vi "Main.vi"(11 "Module Admin":refnum<class "Delacor_lib_QMH_Module Admin.lvclass">) -> ()   [LabVIEW 2020, in "UART Module.lvlib"]
doc: "This template is based off of the Queued Message Handler design pattern and the Queued Message Handler project template that ships with LabVIEW.\n\nThe main difference is that the queue is private to this module and communication between modules is performed via Broadcast and Request events.\n\nRequest events are wrapped in public API methods and are handled in the Event Handling Loop (EHL) of this VI. Any module can register for Broadcast events sent by this module. The EHL generates messages based on user interface actions.\n\nThe Message Handling Loop (MHL) processes messages generated by the EHL, or by other messages. The messages are string values, so new messages can be added easily to the Message Cases case structure in the MHL. Each message cluster can also provide an optional value for Message Data, which is a variant that can be converted to whatever message-specific data is required.\n_____\nBased on DQMH Project Template 7.0.1.1316."
uses:
  UART Module.lvlib
  <vilib>/Delacor/Delacor QMH/Libraries/Module Admin_class/Delacor_lib_QMH_Module Admin.lvclass
  Module Data--cluster.ctl
  Stop Argument--cluster.ctl
  <vilib>/Delacor/Delacor QMH/Libraries/Message Queue_class/Delacor_lib_QMH_Message Queue.lvclass/Delacor_lib_QMH_Message Queue.ctl
  <vilib>/Delacor/Delacor QMH/Libraries/Module Admin_class/Delacor_lib_QMH_Module Admin.lvclass/Delacor_lib_QMH_Module Admin.ctl
  Open Port Argument--cluster.ctl
  Close Port Argument--cluster.ctl
  <vilib>/Utility/miscctls.llb/LVPointTypeDef.ctl
  <vilib>/Delacor/Delacor QMH/Libraries/Message Queue_class/Delacor_lib_QMH_Enqueue Message (Single).vi
  <vilib>/Delacor/Delacor QMH/Libraries/Module Admin_class/Delacor_lib_QMH_Get External Launch.vi
  <vilib>/Delacor/Delacor QMH/Libraries/Message Queue_class/Delacor_lib_QMH_Message Queue.lvclass
  Write Data Argument--cluster.ctl
  checkBufferData Argument--cluster.ctl
  readBuffer Argument--cluster.ctl
  cc7c8281-b699-4288-b638-b774a9bc16a2.vi
  checkBufferSize Argument--cluster.ctl
panel:
  in  "stop":bool
  in  "讀取目標字數":i32=1
  in  "Write":bool
  in  "VISA resource name":refnum<visa-resource-name>
  out "read buffer":string
  in  "write buffer":string
  out "error out":errorcluster
  # "1. 設定 VISA\n2. 設定讀取目標字數\n3. 按下”開始通訊”，進行通訊作業\n4. 設定\"write buffer“\n5. 按下\"Write\"，將資料進行寫入\n6. 觀察\"read buffer\"\n7. 按下停止通訊“，結束通訊作業"
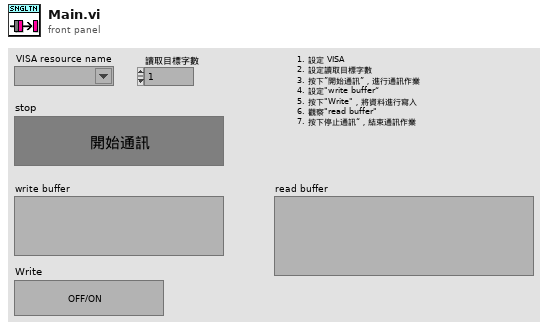
[diagram p1: front panel]
types:
  T1 = typedef "UART Module.lvlib/Request Events--cluster.ctl" = cluster{"Stop Module":refnum<user-event>, "Show Panel":refnum<user-event>, "Hide Panel":refnum<user-event>, "Get Module Execution Status":refnum<user-event>, "Show Diagram":refnum<user-event>, "Open Port":refnum<user-event>, "Close Port":refnum<user-event>, "Write Data":refnum<user-event>, "Private":cluster{"checkBufferData":refnum<user-event>, "readBuffer":refnum<user-event>, "checkBufferSize":refnum<user-event>}}
  T2 = typedef "UART Module.lvlib/Module Data--cluster.ctl" = cluster{"Status":string, "read buffer":string, "VISA":refnum<visa-resource-name>, "targetCount":i32}
  T3 = enum32{"invalid lock state", "Not Locked", "Locked (No Password)", "Password-protected"}
  T4 = typedef "UART Module.lvlib/Stop Argument--cluster.ctl" = cluster{"Origin":string, "Exit via Stop Module Req?":bool, "Wait for Module to stop?":bool}
  T5 = typedef "UART Module.lvlib/Open Port Argument--cluster.ctl" = cluster{"VISA":refnum<visa-resource-name>}
  T6 = typedef "UART Module.lvlib/Close Port Argument--cluster.ctl" = cluster{"Boolean":bool}
  T7 = typedef "UART Module.lvlib/Write Data Argument--cluster.ctl" = cluster{"write data":string}
  T8 = typedef "UART Module.lvlib/checkBufferData Argument--cluster.ctl" = cluster{"Boolean":bool}
  T9 = typedef "UART Module.lvlib/readBuffer Argument--cluster.ctl" = cluster{"Number of Bytes at Serial Port":u32}
  T10 = typedef "UART Module.lvlib/checkBufferSize Argument--cluster.ctl" = cluster{"readBuffer":string}
  T11 = typedef "LVPointTypeDef.ctl" = cluster{"Horizontal":i16, "Vertical":i16}
  T12 = enum32{"Invalid", "Standard", "Closed", "Hidden", "Minimized", "Maximized"}
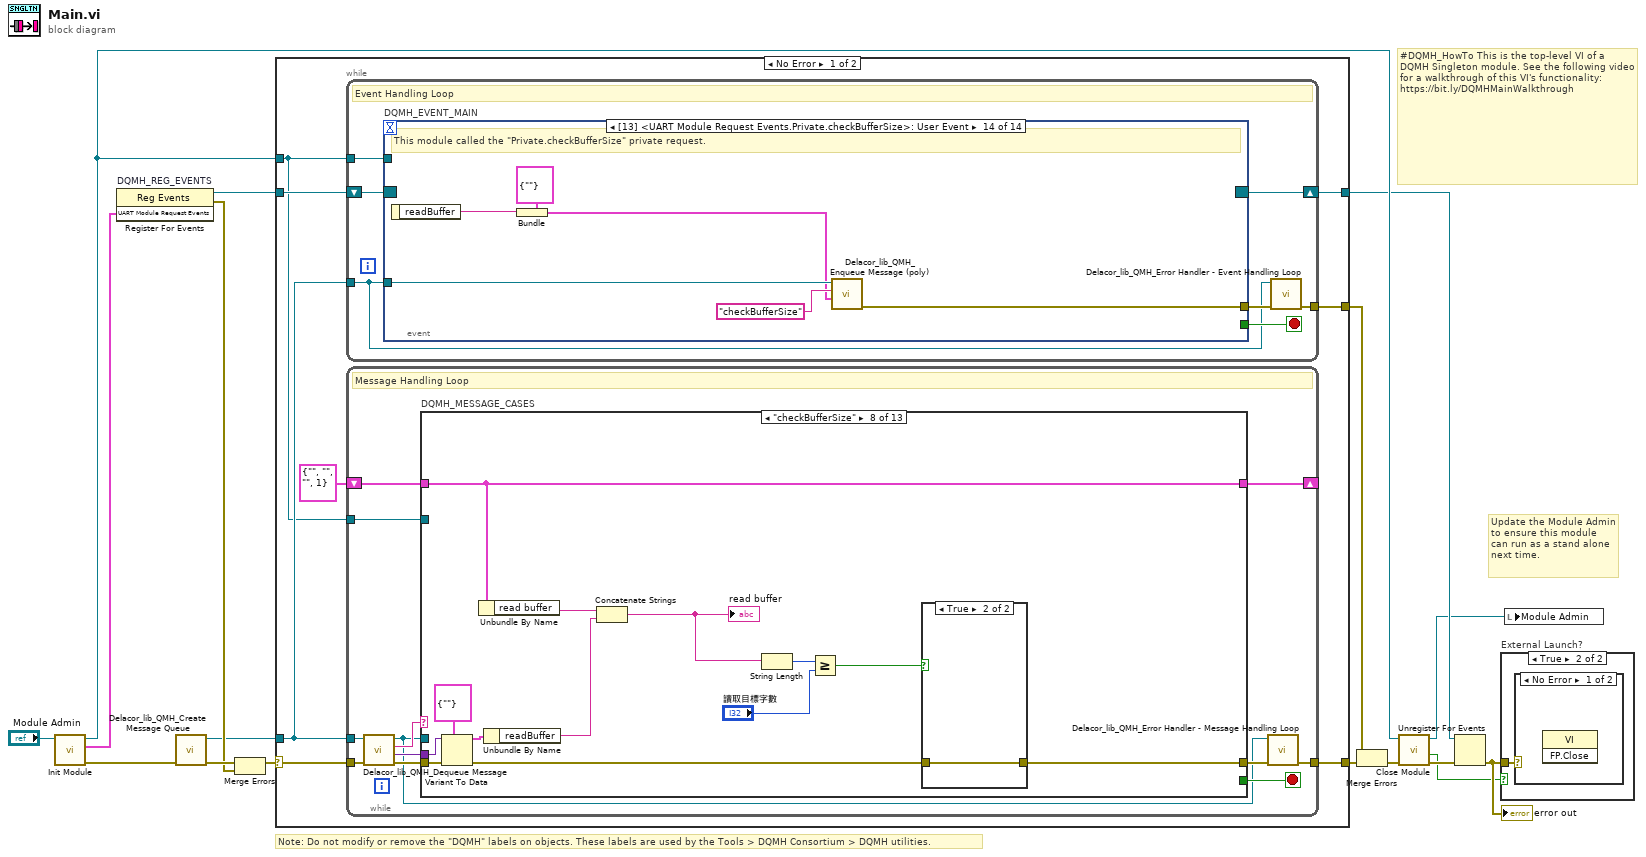
[diagram p0: block diagram]
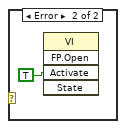
[diagram p3: hidden frame]
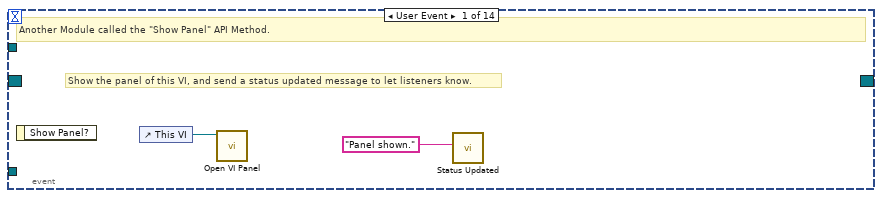
[diagram p4: hidden frame]
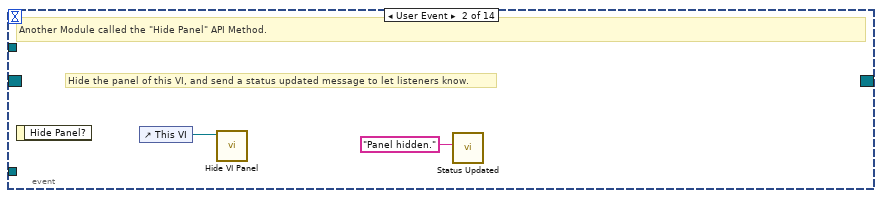
[diagram p5: hidden frame]
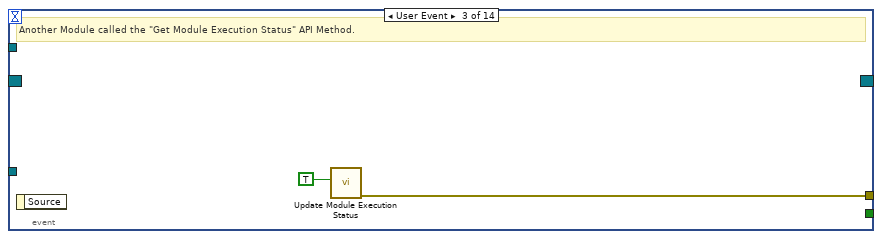
[diagram p6: hidden frame]
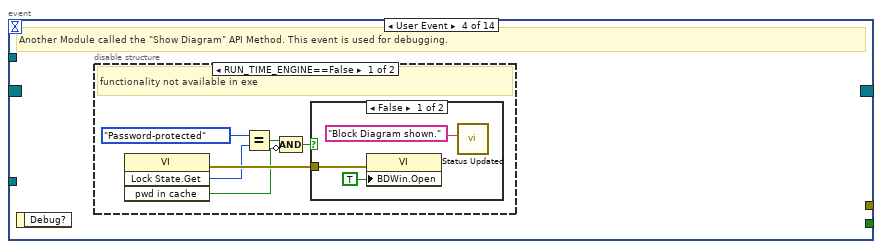
[diagram p7: hidden frame]
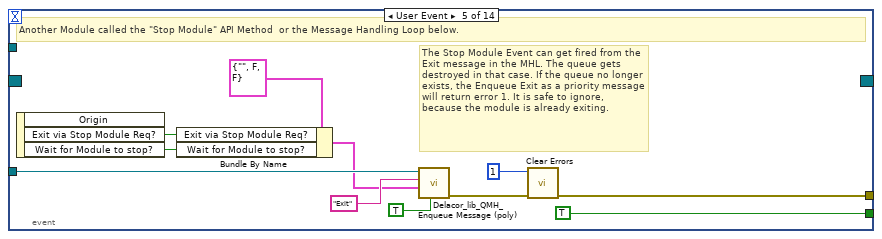
[diagram p10: hidden frame]
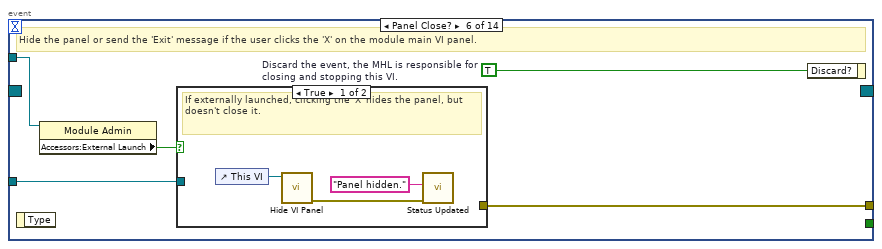
[diagram p11: hidden frame]
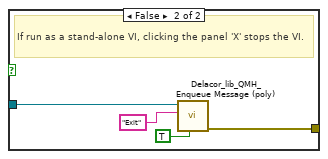
[diagram p12: hidden frame]
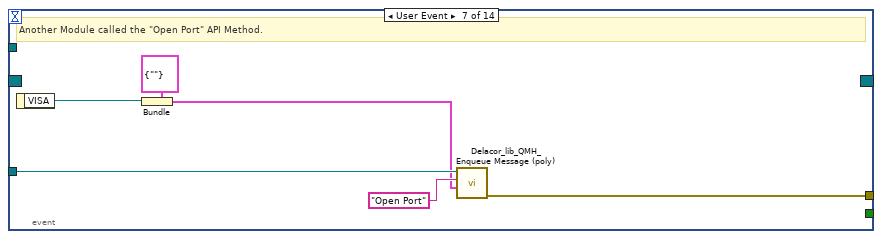
[diagram p13: hidden frame]
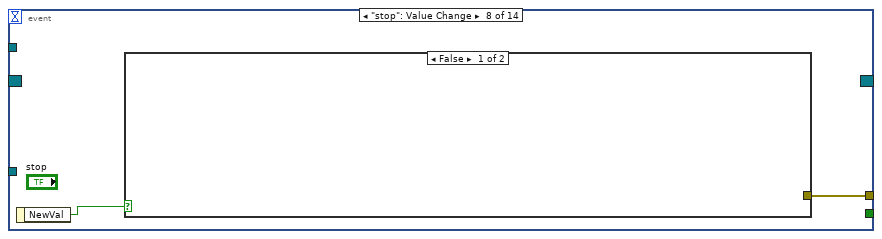
[diagram p14: hidden frame]
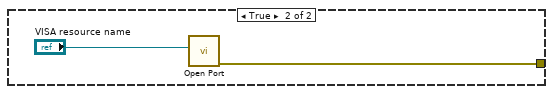
[diagram p15: hidden frame]
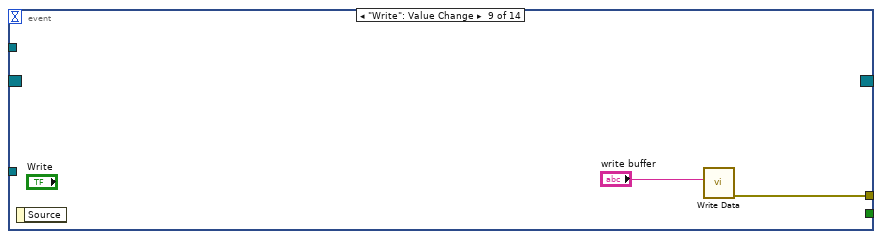
[diagram p16: hidden frame]
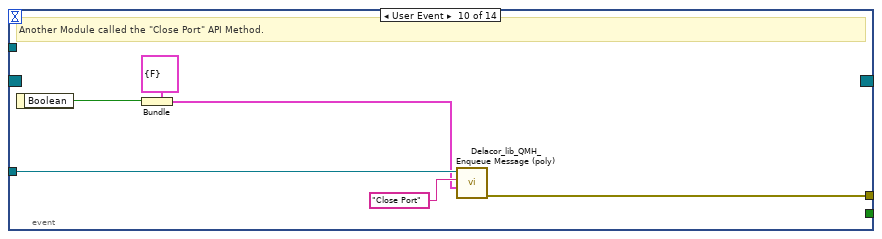
[diagram p17: hidden frame]
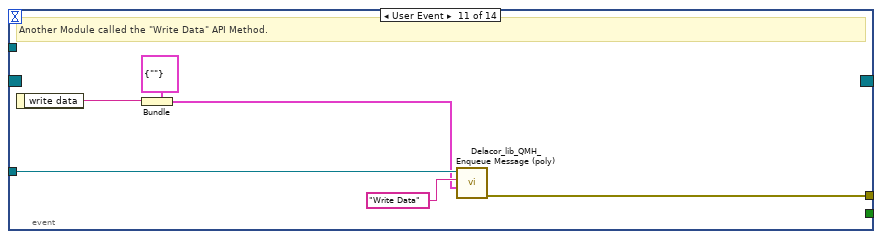
[diagram p18: hidden frame]
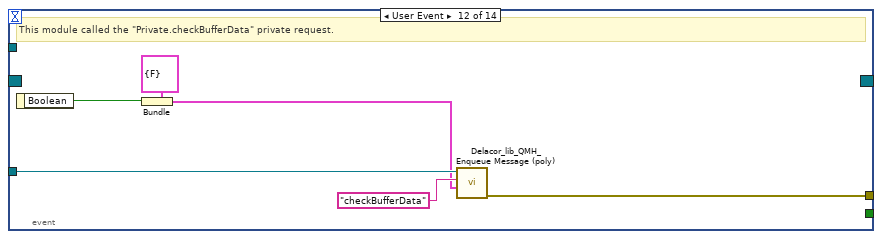
[diagram p19: hidden frame]
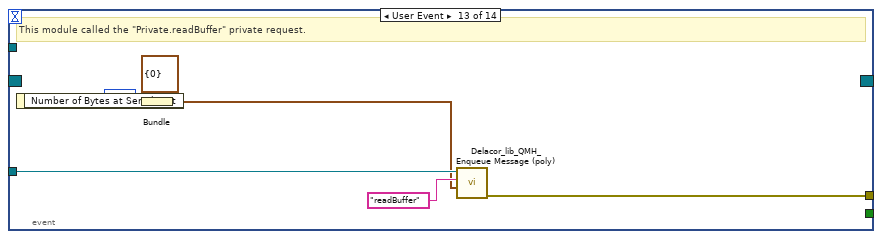
[diagram p20: hidden frame]
diagram:
  # "#DQMH_HowTo This is the top-level VI of a DQMH Singleton module. See the following video for a walkthrough of this VI's functionality: https://bit.ly/DQMHMainWalkthrough"
  # "Note: Do not modify or remove the \"DQMH\" labels on objects. These labels are used by the Tools > DQMH Consortium > DQMH utilities."
  # "Update the Module Admin to ensure this module can run as a stand alone next time."
  n1 = call "Init Module.vi"("Singleton Module Admin in"="Module Admin") -> ("error out"=w16:errorcluster, "UART Module Request Events"=w5:T1, "Singleton Module Admin out"=w8:refnum<class "Delacor_lib_QMH_Module Admin.lvclass">)  [unwired: 8 in]
  n2 = register-events "DQMH_REG_EVENTS"(w5) -> (reference out=w6:refnum<event-registration>, error out=w9:errorcluster)  [unwired: 2 in]
  n3 = call <vilib>:"Delacor_lib_QMH_Create Message Queue.vi"("error in"=w16) -> ("error out"=w11:errorcluster, "Message Queue"=w4:refnum<class "Delacor_lib_QMH_Message Queue.lvclass">)  [unwired: 9 in]
  n4 = Merge Errors(w11, w9) -> (w10:errorcluster)
  n5 = case shown="No Error" w10 {
    selector: w10 -> [w23 w276]
    tunnel: [w25 w275] -> w17
    tunnel: [w22 w274] -> w7
    tunnel: w6 -> [w20 w274]
    tunnel: w4 -> [w19 w269]
    tunnel: [w24 _] -> w14
    tunnel: w8 -> [w18 w270]
    frame No Error {
      n6 = while {
        tunnel: w19 -> [w26]
        shift-right: [w29] -> w22
        shift-left: w20 -> [w30]
        tunnel: [w31] -> w24
        tunnel: w18 -> [w27]
        stop <- w28 stop-if-true
        # "Event Handling Loop"
        n7 = event "DQMH_EVENT_MAIN" shown="[13] <UART Module Request Events.Private.checkBufferSize>: User Event" {
          selector: w30 -> [_ _ _ _ _ _ _ _ _ _ _ _ _ _]
          dyn-events: [_ _ _ _ _ _ _ _ _ _ _ _ _ _] -> w29
          timeout: _ -> [_ _ _ _ _ _ _ _ _ _ _ _ _ _]
          tunnel: [_ _ _ _ TRUE ("Discard?") _ _ _ _ _ _ _ _ _] -> w28
          tunnel: w26 -> [_ _ _ _ w54 w61 w76 _ _ w88 w94 w100 w106 w112]
          tunnel: [_ _ w38 _ w57 w63 w71 w77 w82 w83 w89 w95 w101 w107] -> w32
          tunnel: w27 -> [_ _ _ _ _ w60 _ _ _ _ _ _ _ _]
          event User Event {
            # "Show the panel of this VI, and send a status updated message to let listeners know."
            # "Another Module called the \"Show Panel\" API Method."
            n8 = event-data() -> ()  [unwired: 1 in, 1 out]
            n9 = control-ref of="This VI"() -> (w34:refnum<vi>)
            n10 = call "Open VI Panel.vi"("VI"=w34) -> ()  [unwired: 10 in, 1 out]
            n11 = call "Status Updated.vi"("Status"="Panel shown." ("format string")) -> ()  [unwired: 10 in, 1 out]
          }
          event User Event {
            # "Hide the panel of this VI, and send a status updated message to let listeners know."
            # "Another Module called the \"Hide Panel\" API Method."
            n12 = event-data() -> ()  [unwired: 1 in, 1 out]
            n13 = control-ref of="This VI"() -> (w36:refnum<vi>)
            n14 = call "Hide VI Panel.vi"("VI"=w36) -> ()  [unwired: 10 in, 1 out]
            n15 = call "Status Updated.vi"("Status"="Panel hidden." ("format string")) -> ()  [unwired: 10 in, 1 out]
          }
          event User Event {
            # "Another Module called the \"Get Module Execution Status\" API Method."
            n16 = event-data() -> ()  [unwired: 1 in, 1 out]
            n17 = call "Update Module Execution Status.vi"("Running?"=TRUE) -> ("error out"=w38:errorcluster)  [unwired: 10 in]
          }
          event User Event {
            # "Another Module called the \"Show Diagram\" API Method. This event is used for debugging."
            n18 = event-data() -> ()  [unwired: 1 in, 1 out]
            n19 = disable-structure shown="RUN_TIME_ENGINE==False" {
              frame condition #0 (active) {
                # "functionality not available in exe"
                n20 = invoke on="Invoke Node" class="VI" method="Lock State.Get"() -> (error out=w44:errorcluster, "Get Lock State"=w43:T3, "pwd in cache"=w40:bool)  [unwired: 4 in, 1 out]
                n21 = Equal?(x=T3."Password-protected", y=w43) -> (x = y?=w41:bool)
                n22 = Compound Arithmetic op=AND(w41, invert w40) -> (w39:bool)
                n23 = case shown="False" w39 {
                  tunnel: w44 -> [w47 _]
                  frame False {
                    n24 = property on="Property Node" class="VI"(error in=w47, "BDWin.Open"=TRUE ("Block Diagram Window:Open")) -> ()  [unwired: 1 in, 2 out]
                    n25 = call "Status Updated.vi"("Status"="Block Diagram shown." ("format string")) -> ()  [unwired: 10 in, 1 out]
                  }
                  frame True {
                    # "Password-protected VI, and the password is not in the cache. Do not show the diagram."
                  }
                }
              }
              frame condition #1 {
              }
            }
          }
          event User Event {
            # "The Stop Module Event can get fired from the Exit message in the MHL. The queue gets destroyed in that case. If the queue no longer exists, the Enqueue Exit as a priority message will return error 1. It is safe to ignore, because the module is already exiting."
            # "Another Module called the \"Stop Module\" API Method  or the Message Handling Loop below."
            n26 = event-data() -> ("Exit via Stop Module Req?"=w50:bool, "Wait for Module to stop?"=w49:bool)  [unwired: 1 in, 1 out]
            n27 = Bundle By Name(cluster=T4 {"Origin"="", "Exit via Stop Module Req?"=FALSE, "Wait for Module to stop?"=FALSE} ("Stop Argument"), "Exit via Stop Module Req?"=w50, "Wait for Module to stop?"=w49) -> (w48:T4)
            n28 = call-poly <vilib>:"Delacor_lib_QMH_Enqueue Message (poly).vi"("Priority Message? (F)"=TRUE, "Message Data"=w48, "Message"="Exit", "Message Queue in"=w54) -> ("error out"=w58:errorcluster)  [unwired: 6 in, 1 out]
            n29 = call <vilib>:"Clear Errors.vi"("error in (no error)"=w58, "specific error code to clear (0: all)"=1) -> ("error out"=w57:errorcluster)  [unwired: 4 in, 1 out]
          }
          event Panel Close? {
            w62 = TRUE  # Discard the event, the MHL is responsible for closing and stopping this VI.
            # "Hide the panel or send the 'Exit' message if the user clicks the 'X' on the module main VI panel."
            n30 = event-data() -> ()  [unwired: 1 in, 1 out]
            n31 = property on="Property Node" class="Module Admin"(reference=w60) -> ("Accessors:External Launch"=w59:bool)  [unwired: 1 in, 2 out]
            n32 = case shown="True" w59 {
              tunnel: w61 -> [_ w69]
              tunnel: [_ w70] -> w63
              frame True {
                # "If externally launched, clicking the 'X' hides the panel, but doesn't close it."
                n33 = control-ref of="This VI"() -> (w66:refnum<vi>)
                n34 = call "Hide VI Panel.vi"("VI"=w66) -> ("error out"=w64:errorcluster)  [unwired: 10 in]
                n35 = call "Status Updated.vi"("error in"=w64, "Status"="Panel hidden." ("format string")) -> ()  [unwired: 9 in, 1 out]
              }
              frame False {
                # "If run as a stand-alone VI, clicking the panel 'X' stops the VI."
                n36 = call-poly <vilib>:"Delacor_lib_QMH_Enqueue Message (poly).vi"("Priority Message? (F)"=TRUE, "Message"="Exit", "Message Queue in"=w69) -> ("error out"=w70:errorcluster)  [unwired: 7 in, 1 out]
              }
            }
            n37 = event-data ("Event Filter Node")("Discard?"=w62) -> ()  [unwired: 1 in, 1 out]
          }
          event User Event {
            # "Another Module called the \"Open Port\" API Method."
            n38 = event-data() -> ("VISA"=w72:refnum<visa-resource-name>)  [unwired: 1 in]
            n39 = Bundle(cluster=T5 {"VISA"=""} ("Open Port Argument"), "VISA"=w72) -> (w73:T5)
            n40 = call-poly <vilib>:"Delacor_lib_QMH_Enqueue Message (poly).vi"("Message Data"=w73, "Message"="Open Port", "Message Queue in"=w76) -> ("error out"=w71:errorcluster)  [unwired: 7 in, 1 out]
          }
          event "stop": Value Change {
            n41 = event-data() -> ("NewVal"=w78:bool)  [unwired: 1 in]
            n42 = case shown="False" w78 {
              tunnel: [_ w80] -> w77
              frame False {
              }
              frame True {
                n43 = call "Open Port.vi"("VISA"="VISA resource name") -> ("error out"=w80:errorcluster)  [unwired: 10 in]
              }
            }
          }
          event "Write": Value Change {
            n44 = event-data() -> ()  [unwired: 1 in, 1 out]
            n45 = call "Write Data.vi"("write data"="write buffer") -> ("error out"=w82:errorcluster)  [unwired: 10 in]
          }
          event User Event {
            # "Another Module called the \"Close Port\" API Method."
            n46 = event-data() -> ("Boolean"=w84:bool)  [unwired: 1 in]
            n47 = Bundle(cluster=T6 {"Boolean"=FALSE} ("Close Port Argument"), "Boolean"=w84) -> (w85:T6)
            n48 = call-poly <vilib>:"Delacor_lib_QMH_Enqueue Message (poly).vi"("Message Data"=w85, "Message"="Close Port", "Message Queue in"=w88) -> ("error out"=w83:errorcluster)  [unwired: 7 in, 1 out]
          }
          event User Event {
            # "Another Module called the \"Write Data\" API Method."
            n49 = event-data() -> ("write data"=w90:string)  [unwired: 1 in]
            n50 = Bundle(cluster=T7 {"write data"=""} ("Write Data Argument"), "write data"=w90) -> (w91:T7)
            n51 = call-poly <vilib>:"Delacor_lib_QMH_Enqueue Message (poly).vi"("Message Data"=w91, "Message"="Write Data", "Message Queue in"=w94) -> ("error out"=w89:errorcluster)  [unwired: 7 in, 1 out]
          }
          event User Event {
            # "This module called the \"Private.checkBufferData\" private request."
            n52 = event-data() -> ("Boolean"=w96:bool)  [unwired: 1 in]
            n53 = Bundle(cluster=T8 {"Boolean"=FALSE} ("checkBufferData Argument"), "Boolean"=w96) -> (w97:T8)
            n54 = call-poly <vilib>:"Delacor_lib_QMH_Enqueue Message (poly).vi"("Message Data"=w97, "Message"="checkBufferData", "Message Queue in"=w100) -> ("error out"=w95:errorcluster)  [unwired: 7 in, 1 out]
          }
          event User Event {
            # "This module called the \"Private.readBuffer\" private request."
            n55 = event-data() -> ("Number of Bytes at Serial Port"=w102:u32)  [unwired: 1 in]
            n56 = Bundle(cluster=T9 {"Number of Bytes at Serial Port"=0} ("readBuffer Argument"), "Number of Bytes at Serial Port"=w102) -> (w103:T9)
            n57 = call-poly <vilib>:"Delacor_lib_QMH_Enqueue Message (poly).vi"("Message Data"=w103, "Message"="readBuffer", "Message Queue in"=w106) -> ("error out"=w101:errorcluster)  [unwired: 7 in, 1 out]
          }
          event User Event {
            # "This module called the \"Private.checkBufferSize\" private request."
            n58 = event-data() -> ("readBuffer"=w108:string)  [unwired: 1 in]
            n59 = Bundle(cluster=T10 {"readBuffer"=""} ("checkBufferSize Argument"), "readBuffer"=w108) -> (w109:T10)
            n60 = call-poly <vilib>:"Delacor_lib_QMH_Enqueue Message (poly).vi"("Message Data"=w109, "Message"="checkBufferSize", "Message Queue in"=w112) -> ("error out"=w107:errorcluster)  [unwired: 7 in, 1 out]
          }
        }
        n61 = call-dynamic "Delacor_lib_QMH_Error Handler - Event Handling Loop.vi"("error in"=w32, "Message Queue in"=w26) -> ("dup error in"=w31:errorcluster)  [unwired: 8 in, 1 out]
      }
      n62 = while {
        tunnel: w19 -> [w113]
        shift-right: [w121] -> _
        shift-left: T2 {"Status"="", "read buffer"="", "VISA"="", "targetCount"=1} ("Data Cluster") -> [w122]
        tunnel: w23 -> [w124]
        tunnel: [w116] -> w25
        tunnel: w18 -> [w117]
        stop <- w120 stop-if-true
        # "Message Handling Loop"
        n63 = call-dynamic "Delacor_lib_QMH_Dequeue Message.vi"("error in"=w124, "Message Queue in"=w113) -> ("error out"=w123:errorcluster, "Message Data"=w118:variant, "Message"=w119:string, "Message Queue out"=w114:refnum<class "Delacor_lib_QMH_Message Queue.lvclass">)  [unwired: 6 in]
        n64 = case "DQMH_MESSAGE_CASES" shown="\"checkBufferSize\"" w119 {
          selector: w119 -> [_ _ _ _ _ _ _ _ _ _ _ _ w264]
          tunnel: w114 -> [_ _ _ _ _ _ _ _ _ _ w230 w252 _]
          tunnel: w123 -> [w142 w146 w161 w168 w178 w187 w205 w218 w224 w226 w237 w258 w267]
          tunnel: [w140 w146 w148 w167 w169 w180 w196 w213 w223 w226 w233 w253 w268] -> w115
          tunnel: w122 -> [w131 w145 w149 w163 w173 w182 w199 w212 w222 w225 w232 w251 w265]
          tunnel: [w130 w145 w150 w163 w173 w182 w199 w212 w222 w225 w232 w251 w265] -> w121
          tunnel: [_ _ _ _ _ _ _ _ _ _ _ w250 _] -> w120
          tunnel: w118 -> [_ _ w160 w166 w176 w186 w204 w217 _ _ w231 w249 _]
          tunnel: w117 -> [w132 _ _ _ _ _ _ _ _ _ w229 w244 _]
          frame "Initialize" {
            # "#CodeNeeded - Initialize the appearance of the front panel."
            # "#CodeNeeded - Initialize your state data here."
            # "Initialize - Any operation that needs to be done before the module can receive messages. Synchronize Caller Events.vi will inform Start Module.vi that the module has launched and is ready to receive messages. Module Did Init.vi will broadcast that the module initialized."
            n65 = call "Synchronize Caller Events.vi"("error in"=w142, "Singleton Module Admin in"=w132) -> ("error out"=w141:errorcluster, "Singleton Module Admin out"=w127:refnum<class "Delacor_lib_QMH_Module Admin.lvclass">)  [unwired: 8 in]
            n66 = property on="Property Node" class="Module Admin"(reference=w127) -> ("Accessors:External Launch"=w136:bool)  [unwired: 1 in, 2 out]
            n67 = Select(t=T12."Hidden" ("State"), s=w136, f=T12."Standard" ("State")) -> (s? t:f=w133:T12)
            n68 = call "Module Name--constant.vi"() -> ("Module Name"=w139:string)  [unwired: 11 in]
            n69 = property on="Property Node" class="VI"("Front Panel.Title"=w139) -> (reference out=w138:refnum<vi>, error out=w144:errorcluster)  [unwired: 2 in]
            n70 = call "Module Name--constant.vi"() -> ("Module Name"=w128:string)  [unwired: 11 in]
            n71 = invoke on="Invoke Node" class="VI" method="FP.Open"(reference=w138, error in=w144, "State"=w133) -> (reference out=w137:refnum<vi>, error out=w143:errorcluster)  [unwired: 2 in, 3 out]
            n72 = Bundle By Name(cluster=w131, "Status"="Initial Message" ("Initial Message")) -> (w130:T2)
            n73 = call "Module Did Init.vi"("error in"=w141, "Initialized?"=TRUE, "Origin"=w128) -> ("error out"=w140:errorcluster)  [unwired: 8 in]
            n74 = invoke on="Invoke Node" class="VI" method="FP.Center"(reference=w137, error in=w143) -> ()  [unwired: 1 in, 3 out]
            n75 = property on="Pane" class="Pane"("Origin"=T11 {"Horizontal"=0, "Vertical"=0}) -> ()  [unwired: 2 in, 2 out]
          }
          frame "---Module Specific---" {
            # "Separator -- The following cases handle messages specific to this Module."
          }
          frame "Open Port" {
            w153 = u16 0 items=["None", "Last Bit", "TermChar", "Break"] ("Serial Settings:End Mode for Writes")
            w155 = u16 0 items=["None", "Last Bit", "TermChar"] ("Serial Settings:End Mode for Reads")
            n76 = Variant To Data(error in=w161, type=T5 {"VISA"=""} ("Open Port Argument"), Variant=w160) -> (data=w158:T5, error out=w152:errorcluster)
            n77 = Unbundle By Name(w158) -> ("VISA"=w151:refnum<visa-resource-name>)
            n78 = VISA Open(error in (no error)=w152, VISA resource name=w151) -> (VISA resource name=w157:refnum<visa-resource-name>, error out=w156:errorcluster)  [unwired: 3 in]
            n79 = property class="Instr"(reference=w157, error in=w156, "ASRL End In"=w155, "ASRL End Out"=w153) -> (reference out=w154:refnum<visa-resource-name>, error out=w147:errorcluster)
            n80 = Merge Errors(w147) -> (w148:errorcluster)
            n81 = Bundle By Name(cluster=w149, "VISA"=w154) -> (w150:T2)
          }
          frame "Close Port" {
            n82 = Variant To Data(error in=w168, type=T6 {"Boolean"=FALSE} ("Close Port Argument"), Variant=w166) -> (data=w164:T6, error out=w167:errorcluster)
            n83 = Unbundle By Name(w164) -> ()  [unwired: 1 out]
            n84 = Unbundle By Name(w163) -> ("VISA"=w162:refnum<visa-resource-name>)
            n85 = VISA Close(VISA resource name=w162) -> ()  [unwired: 1 in, 1 out]
          }
          frame "Write Data" {
            n86 = Variant To Data(error in=w178, type=T7 {"write data"=""} ("Write Data Argument"), Variant=w176) -> (data=w174:T7, error out=w177:errorcluster)
            n87 = Unbundle By Name(w174) -> ("write data"=w171:string)
            n88 = Unbundle By Name(w173) -> ("VISA"=w172:refnum<visa-resource-name>)
            n89 = VISA Write(VISA resource name=w172, write buffer=w171, error in (no error)=w177) -> (error out=w170:errorcluster)  [unwired: 2 out]
            n90 = call "checkBufferData.vi"("error in"=w170) -> ("error out"=w169:errorcluster)  [unwired: 10 in]
          }
          frame "checkBufferData" {
            n91 = Variant To Data(error in=w187, type=T8 {"Boolean"=FALSE} ("checkBufferData Argument"), Variant=w186) -> (data=w184:T8, error out=w181:errorcluster)
            n92 = Unbundle By Name(w184) -> ()  [unwired: 1 out]
            n93 = Unbundle By Name(w182) -> ("VISA"=w183:refnum<visa-resource-name>)
            n94 = property class="Instr"(reference=w183) -> ("Bytes at Port"=w179:u32)  [unwired: 1 in, 2 out]
            n95 = case shown="0, Default" w179 {
              selector: w179 -> [_ w192]
              tunnel: w181 -> [w191 w194]
              tunnel: [w188 w193] -> w180
              frame 0, Default {
                n96 = call "Stall Data Flow.vim"("value in"=w191, "milliseconds to wait"=u32 200) -> ("value out"=w189:errorcluster)  [unwired: 1 out]
                n97 = call "checkBufferData.vi"("error in"=w189) -> ("error out"=w188:errorcluster)  [unwired: 10 in]
              }
              frame 1.. {
                n98 = call "readBuffer.vi"("error in"=w194, "Number of Bytes at Serial Port"=w192) -> ("error out"=w193:errorcluster)  [unwired: 9 in]
              }
            }
          }
          frame "readBuffer" {
            n99 = Variant To Data(error in=w205, type=T9 {"Number of Bytes at Serial Port"=0} ("readBuffer Argument"), Variant=w204) -> (data=w202:T9, error out=w200:errorcluster)
            n100 = Unbundle By Name(w202) -> ("Number of Bytes at Serial Port"=w201:u32)
            n101 = Unbundle By Name(w199) -> ("VISA"=w198:refnum<visa-resource-name>)
            n102 = VISA Read(VISA resource name=w198, byte count=w201, error in (no error)=w200) -> (read buffer=w195:string, error out=w197:errorcluster)  [unwired: 2 out]
            n103 = call "checkBufferSize.vi"("error in"=w197, "readBuffer"=w195) -> ("error out"=w196:errorcluster)  [unwired: 9 in]
          }
          frame "checkBufferSize" {
            n104 = Variant To Data(error in=w218, type=T10 {"readBuffer"=""} ("checkBufferSize Argument"), Variant=w217) -> (data=w215:T10, error out=w214:errorcluster)
            n105 = Unbundle By Name(w212) -> ("read buffer"=w211:string)
            n106 = Unbundle By Name(w215) -> ("readBuffer"=w210:string)
            n107 = Concatenate Strings(w211, w210) -> (w208:string)
            "read buffer" <- w208
            n108 = String Length(string=w208) -> (length=w209:i32)
            n109 = Greater Or Equal?(x=w209, y="讀取目標字數") -> (x >= y?=w206:bool)
            n110 = case shown="True" w206 {
              tunnel: w214 -> [w220 w221]
              tunnel: [w219 w221] -> w213
              frame False {
                n111 = call "checkBufferData.vi"("error in"=w220) -> ("error out"=w219:errorcluster)  [unwired: 10 in]
              }
              frame True {
              }
            }
          }
          frame "---Copy This Frame---" {
            # "Duplicate this frame when creating new messages.  Change this comment in the duplicated frame to describe this message."
            n112 = Merge Errors(w224) -> (w223:errorcluster)
          }
          frame "---Exit and Error Handling---" {
            # "Separator - The following cases handle errors and exit messages."
          }
          frame "Error" {
            # "#CodeRecommended - If the module is running in standalone mode (External Launch = FALSE), this code will pop up an error dialog and call the 'Exit' message if an error occurs. Add more fine-grained error management here."
            # "Error - Check the error message data and respond accordingly. This message is sent by the \"Error Handler\" VIs at the end of each loop in this application."
            n113 = property on="Property Node" class="Module Admin"(reference=w229) -> ("Accessors:External Launch"=w228:bool)  [unwired: 1 in, 2 out]
            n114 = Variant To Data(error in=w237, type=errorcluster {"status"=FALSE, "code"=0, "source"=""} ("error constant"), Variant=w231) -> (data=w227:errorcluster, error out=w235:errorcluster)
            n115 = local write "error out"(w227) -> ()
            n116 = call "Error Reported.vi"("Error"=w227) -> ()  [unwired: 10 in, 1 out]
            n117 = case shown="False" w228 {
              tunnel: [w242 _] -> w234
              tunnel: w230 -> [w240 _]
              tunnel: w227 -> [w241 _]
              frame False {
                n118 = disable-structure shown="Default" {
                  disable-tunnel: w241 -> [w243 _]
                  frame condition #0 (active) {
                    # "If the module is running standalone, then pop up an error dialog and call the \"Exit\" message."
                    n119 = call <vilib>:"Simple Error Handler.vi"("error in (no error)"=w243) -> ()  [unwired: 4 in, 5 out]
                  }
                  frame condition #1 {
                    # "To prevent the Simple Error Handler VI from being loaded (e.g. when deploying to a Real-Time target), add the Conditional Disable Symbol \"DQMH_Disable_SEH\" to your project and set it to TRUE."
                  }
                }
                n120 = call-poly <vilib>:"Delacor_lib_QMH_Enqueue Message (poly).vi"("Priority Message? (F)"=TRUE, "Message"="Exit", "Message Queue in"=w240) -> ("error out"=w242:errorcluster)  [unwired: 7 in, 1 out]
              }
              frame True {
                # "If the module was launched externally, calling the Error Reported broadcast VI is the only action performed by the \"Error\" message. The module's caller can then process the error appropriately."
              }
            }
            n121 = Merge Errors(w235, w234) -> (w233:errorcluster)
          }
          frame "Exit" {
            w248 = 91  # 91: not all Exit messages will have an argument
            w250 = TRUE  # Stop the VI
            # "Release the message queue reference"
            # "#CodeNeeded - Add any required cleanup code here."
            # "Exit - Exit the application."
            n122 = Variant To Data(error in=w258, type=T4 {"Origin"="", "Exit via Stop Module Req?"=FALSE, "Wait for Module to stop?"=FALSE} ("Stop Argument"), Variant=w249) -> (data=w246:T4, error out=w255:errorcluster)
            n123 = call <vilib>:"Clear Errors.vi"("error in (no error)"=w255, "specific error code to clear (0: all)"=w248) -> ("error out"=w257:errorcluster)  [unwired: 4 in, 1 out]
            n124 = control-ref of="This VI"() -> (w245:refnum<vi>)
            n125 = call-dynamic "Delacor_lib_QMH_Release Message Queue.vi"("error in"=w257, "Message Queue"=w252) -> ("error out"=w256:errorcluster)  [unwired: 9 in]
            n126 = call "Handle Exit.vi"("Stop Argument"=w246, "Admin in"=w244, "VI reference"=w245) -> ("error out"=w254:errorcluster)  [unwired: 7 in, 1 out]
            n127 = Merge Errors(w256, w254) -> (w253:errorcluster)
            n128 = call "Error Reported.vi"("Error"=w253) -> ()  [unwired: 10 in, 1 out]
          }
          frame Default {
            # "'Default' case only runs if there is a message that isn't defined in any of the other cases.  Output a programming error."
            n129 = call "Module Name--constant.vi"() -> ("Module Name"=w263:string)  [unwired: 11 in]
            n130 = Format Into String(format string="The invalid message string \"%s\" was received in the Message Handling Loop for module \"%s\".", w264, w263) -> (resulting string=w259:string)  [unwired: 2 in, 1 out]
            n131 = call <vilib>:"Error Cluster From Error Code.vi"("show call chain? (False)"=TRUE, "error message (\"\")"=w259, "error code (0)"=1) -> ("error out"=w266:errorcluster)  [unwired: 6 in]
            n132 = Merge Errors(w267, w266) -> (w268:errorcluster)
          }
        }
        n133 = call-dynamic "Delacor_lib_QMH_Error Handler - Message Handling Loop.vi"("error in"=w115, "Message Queue in"=w114) -> ("dup error in"=w116:errorcluster)  [unwired: 8 in, 1 out]
      }
    }
    frame Error {
      # "Synchronize Caller Events.vi will inform Start Module.vi that the module has launched and will let the code calling Start Module.vi register for broadcasts and would permit the caller receive the broadcast that an error occurred at launch time."
      n134 = call-dynamic "Delacor_lib_QMH_Release Message Queue.vi"("error in"=w276, "Message Queue"=w269) -> ("error out"=w275:errorcluster)  [unwired: 9 in]
      n135 = call "Synchronize Caller Events.vi"("Singleton Module Admin in"=w270) -> ("error out"=w277:errorcluster)  [unwired: 9 in, 1 out]
      n136 = call "Module Name--constant.vi"() -> ("Module Name"=w273:string)  [unwired: 11 in]
      n137 = Format Into String(format string="An error occurred during initialization. %s is no longer running.", w273) -> (resulting string=w271:string)  [unwired: 2 in, 1 out]
      n138 = Merge Errors(w275, w277) -> (w278:errorcluster)
      n139 = call "Error Reported.vi"("Additional Information"=w271, "Error"=w278) -> ()  [unwired: 9 in, 1 out]
    }
  }
  n140 = Merge Errors(w14, w17) -> (w13:errorcluster)
  n141 = call "Close Module.vi"("error in"=w13, "Module Admin in"=w8) -> ("error out"=w15:errorcluster, "External Launch"=w1:bool, "Module Admin out"=w2:refnum<class "Delacor_lib_QMH_Module Admin.lvclass">)  [unwired: 7 in]
  n142 = Unregister For Events(event registration refnum=w7, error in=w15) -> (error out=w12:errorcluster)
  "error out" <- w12
  n143 = case "External Launch?" shown="True" w1 {
    tunnel: w12 -> [_ w279]
    frame False {
    }
    frame True {
      n144 = case shown="No Error" w279 {
        frame No Error {
          n145 = invoke on="Invoke Node" class="VI" method="FP.Close"() -> ()  [unwired: 3 in, 3 out]
        }
        frame Error {
          n146 = invoke on="Invoke Node" class="VI" method="FP.Open"("Activate"=TRUE ("Activate?")) -> ()  [unwired: 4 in, 5 out]
        }
      }
    }
  }
  n147 = local write "Module Admin"(w2) -> ()
